vi "Is Network.vi"(10 "Connection":set{string}(c389), 11 "Proto in":refnum<class "Proto.lvclass">) -> (2 "nerwork?":bool, 3 "Proto out":refnum<class "Proto.lvclass">)   [LabVIEW 2020, in "Proto.lvclass"]
uses:
  Proto.lvclass
  Proto.lvclass/Proto.ctl
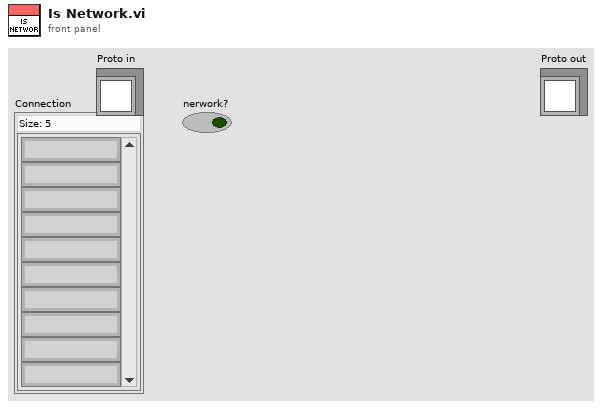
[diagram p1: front panel]
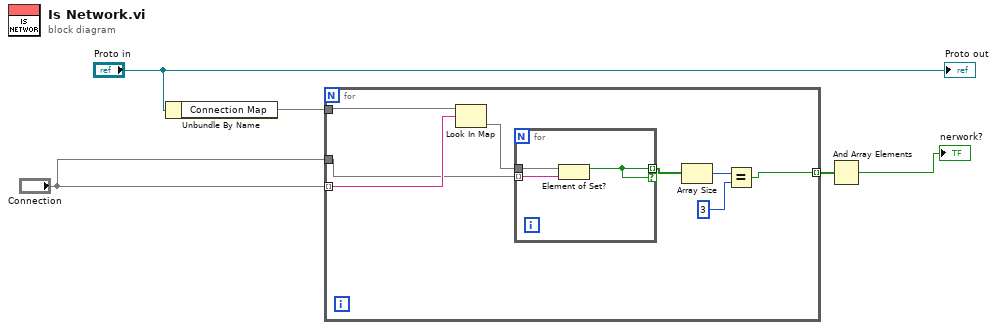
[diagram p0: block diagram]
diagram:
  n1 = Unbundle By Name("Proto in") -> ("Connection Map"=w4:map{string, set{string}})
  n2 = for {
    tunnel: "Connection" -> [w12] mode=indexing
    tunnel: w4 -> [w13]
    tunnel: "Connection" -> [w10]
    tunnel: [w7] -> w3 mode=indexing
    n3 = Look In Map(map=w13, key=w12) -> (value=w11:set{string})  [unwired: 1 in, 1 out]
    n4 = for {
      tunnel: w11 -> [w16]
      tunnel: w10 -> [w15] mode=indexing
      tunnel: [w14] -> w9 mode=indexing if=w14
      n5 = Element of Set?(10:w15, 11:w16) -> (3:w14:bool)
    }
    n6 = Array Size(array=w9) -> (size(s)=w8:i32)
    n7 = Equal?(x=w8, y=3) -> (x = y?=w7:bool)
  }
  n8 = And Array Elements(Boolean array=w3) -> (logical AND=→"nerwork?":bool)
  "Proto out" <- "Proto in"
